vi "Run_Async.vi"(8 "error in":errorcluster, 10 "Core Number":u16=1 min=1 step=1, 11 "Port Number":u16=1444) -> (0 "error out":errorcluster, 2 "Response From Server":string, 3 "Pass?":bool)   [LabVIEW 2019]
uses:
  <userlib>/_TI-LA/Reusable/CCS/APIs/CCS.lvlib
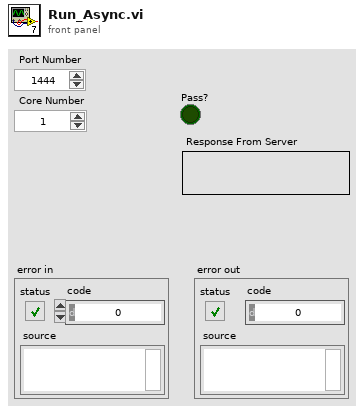
[diagram p1: front panel]
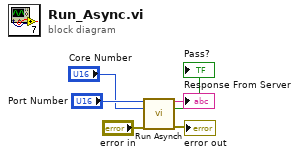
[diagram p0: block diagram]
diagram:
  n1 = call <userlib>:"Run Asynch.vi"("Port Number"="Port Number", "Core Number"="Core Number", "error in"="error in") -> ("Response From Server"=→"Response From Server":string, "Pass?"=→"Pass?":bool, "error out"=→"error out":errorcluster)  [unwired: 10 in]
